vi "TREE_FGV_List Symbol.vi"(6 "Oper":enum16{"Initial", "Get Symbol", "Clear"}(ring)=enum."Get Symbol", 7 "Control":refnum<vi>, 9 "Symbol":i32, 10 "Picture Name":string) -> (1 "Symbol Index":i32)   [LabVIEW 2016]
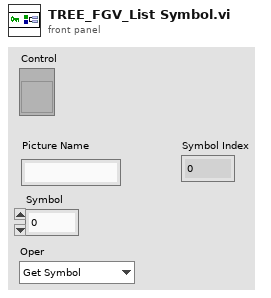
[diagram p1: front panel]
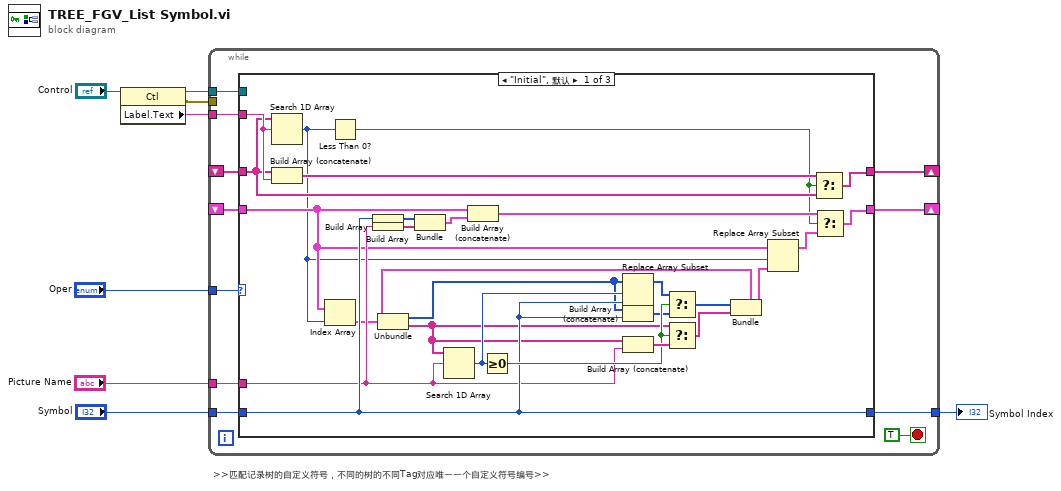
[diagram p0: block diagram]
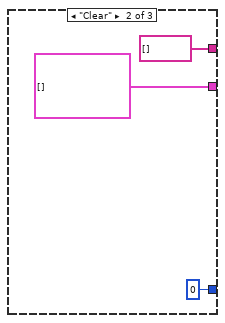
[diagram p2: hidden frame]
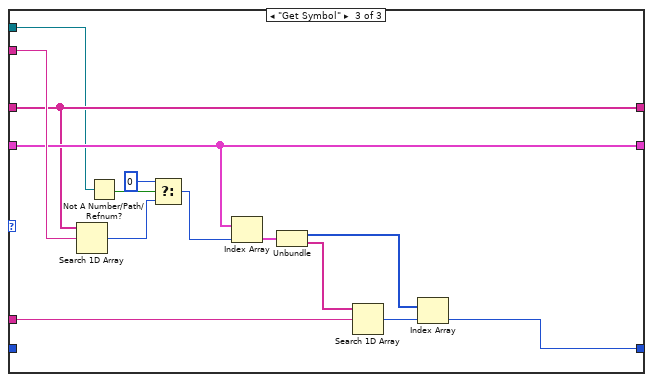
[diagram p3: hidden frame]
diagram:
  # ">>匹配记录树的自定义符号，不同的树的不同Tag对应唯一一个自定义符号编号>>"
  n1 = property class="Ctl"(reference="Control") -> (reference out=w1:refnum<vi>, error out=w3:errorcluster, "Label.Text"=w2:string)  [unwired: 1 in]
  n2 = while {
    tunnel: "Oper" -> [w19]
    tunnel: "Picture Name" -> [w18]
    tunnel: [w16] -> w6
    tunnel: "Symbol" -> [w15]
    shift-right: [w10] -> _
    shift-left: _ -> [w14]
    shift-right: [w11] -> _
    shift-left: _ -> [w12]
    tunnel: w2 -> [w13]
    tunnel: w3 -> [_]
    tunnel: w1 -> [w9]
    stop <- TRUE stop-if-true
    n3 = case shown="\"Initial\", 默认" w19 {
      tunnel: w18 -> [w36 _ w58]
      tunnel: [w37 0 ("Symbol") w54] -> w16
      tunnel: w15 -> [w37 _ _]
      tunnel: w14 -> [w38 _ w55]
      tunnel: w13 -> [w40 _ w61]
      tunnel: w12 -> [w27 _ w56]
      tunnel: [w21 cluster{i32[], string[]}[] [] w56] -> w11
      tunnel: [w20 string[] [] w55] -> w10
      tunnel: w9 -> [_ _ w53]
      frame "Initial", Default {
        n4 = Search 1D Array(1D array=w38, element=w40) -> (index of element=w25:i32)  [unwired: 1 in]
        n5 = Build Array (concatenate)(w38, w40) -> (w39:string[])
        n6 = Index Array(array=w27, index=w25) -> (element=w30:cluster{i32[], string[]})
        n7 = Less Than 0?(x=w25) -> (x < 0?=w22:bool)
        n8 = Build Array(w37) -> (w34:i32[])
        n9 = Build Array(w36) -> (w35:string[])
        n10 = Unbundle(w30) -> (w32:i32[], w31:string[])
        n11 = Bundle(w34, w35) -> (w33:cluster{i32[], string[]})  [unwired: 1 in]
        n12 = Search 1D Array(1D array=w31, element=w36) -> (index of element=w45:i32)  [unwired: 1 in]
        n13 = Build Array (concatenate)(w27, w33) -> (w24:cluster{i32[], string[]}[])
        n14 = Greater Or Equal To 0?(x=w45) -> (x >= 0?=w43:bool)
        n15 = Replace Array Subset(array=w32, new element=w37, index=w45) -> (w42:i32[])
        n16 = Build Array (concatenate)(w32, w37) -> (w41:i32[])
        n17 = Build Array (concatenate)(w31, w36) -> (w44:string[])
        n18 = Select(t=w42, s=w43, f=w41) -> (s? t:f=w29:i32[])
        n19 = Select(t=w31, s=w43, f=w44) -> (s? t:f=w28:string[])
        n20 = Bundle(cluster=w30, w29, w28) -> (w26:cluster{i32[], string[]})
        n21 = Replace Array Subset(array=w27, new element=w26, index=w25) -> (w23:cluster{i32[], string[]}[])
        n22 = Select(t=w39, s=w22, f=w38) -> (s? t:f=w20:string[])
        n23 = Select(t=w24, s=w22, f=w23) -> (s? t:f=w21:cluster{i32[], string[]}[])
      }
      frame "Clear" {
      }
      frame "Get Symbol" {
        n24 = Search 1D Array(1D array=w55, element=w61) -> (index of element=w51:i32)  [unwired: 1 in]
        n25 = Not A Number/Path/Refnum?(number/path/refnum=w53) -> (NaN/Path/Refnum?=w52:bool)
        n26 = Select(t=0, s=w52, f=w51) -> (s? t:f=w49:i32)
        n27 = Index Array(array=w56, index=w49) -> (element=w60:cluster{i32[], string[]})
        n28 = Unbundle(w60) -> (w57:i32[], w59:string[])
        n29 = Search 1D Array(1D array=w59, element=w58) -> (index of element=w62:i32)  [unwired: 1 in]
        n30 = Index Array(array=w57, index=w62) -> (element=w54:i32)
      }
    }
  }
  "Symbol Index" <- w6
